vi "SVT Get Spectrum Subset.vi"   [LabVIEW 2017]
doc: "Extracts the subset of the spectrum specified by <B>frequency range</B>. f0 is updated to reflect the new start frequency, df is the same as in the input spectrum, and the spectrum array is shortened so the last element corresponds with the stop frequency specified in the <B>frequency range</B>. Use this VI for operations such as limiting subsequent frequency operations to the region of interest or removing the part of the spectrum outside the alias-free bandwidth, as well as others."
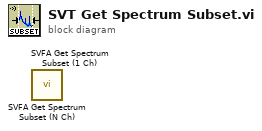
[diagram p0: block diagram]
diagram:
  n1 = call <vilib>:"SVFA Get Spectrum Subset (N Ch).vi"() -> ()  [unwired: 14 in, 6 out]
  n2 = call <vilib>:"SVFA Get Spectrum Subset (1 Ch).vi"() -> ()  [unwired: 14 in, 6 out]
